vi "Test_DIGIT_5122_Standalone.vi"(8 "error in (no error)":errorcluster, 11 "Use Software Trigger":bool=TRUE) -> (0 "error out":errorcluster)   [LabVIEW 2015]
doc: "This VI inits a waveform generation session for AWG-5421. This is a basic example that shows how to setup the board in order to generate waveforms according to a script. \nBy default this configuration uses one channel CH0, and one script trigger ScriptTrigger0. The ScriptTrigger0 is waiting for an external trigger : i.e. a digital Edge on pin PFI 0 by default.\n\nThere are various options for the script to be used. Consult the Script control help for more information on configuring the example for specific scripts."
uses:
  controls/DIGIT_5122_Inputs.ctl
  <instrlib>/niScope/Controls/niScope trigger source.ctl
  controls/DATA_Inputs.ctl
  controls/SOFTWARE_Inputs.ctl
  <instrlib>/niScope/Configure/Trigger/niScope Configure Trigger Edge.vi
  <instrlib>/niScope/Configure/Trigger/niScope Configure Trigger Immediate.vi
  <instrlib>/niScope/Acquire/Fetch/niScope Multi Fetch Binary 16.vi
panel:
  out "wfm info":T1(array[cluster])
  in  "Number of Acquisitions":i32=2
  in  "Accum Number":i16
  out "ASCII Character":string="T"
  in  "SOFTWARE Inputs":T2={"Application Directory"=path "D:/S.O.F.T.S/LABVIEW/PIL", "Data Path"=path "D:/PIRENEA/DATA", "XML Path"=path "D:/PIRENEA/DATA", "XML File Filter"="*.xml", "XML Saved Path"=path "D:/S.O.F.T.S/LABVIEW/PIL/resources", "Excit Scripts Path"=path "D:/PIRENEA/EXCIT_SCRIPTS", "Excit Scripts File Filter"="*.txt", "Excit Waveforms Path"=path "D:/PIRENEA/EXCIT_WFMS", "Excit Waveforms File Filter"="*.bin", "Timing Scripts Path"=path "D:/PIRENEA/TIMING_SCRIPTS", "Timing Scripts File Filter"="*.txt", "Timing Waveforms Path"=path "D:/PIRENEA/TIMING_WFMS", "Timing Waveforms File Filter"="*.bin", "Trapping Waveforms Path"=path "D:/PIRENEA/TRAPPING_WFMS", "Trapping Waveforms File Filter"="*.bin"} caption="EXCIT Paths"
  out "Graphe":ext[][](graph)
  out "acquisition status":i32
  in  "DATA Inputs":T3={"Record Length"=100000, "Sample Rate"=10000000.0, "Data Type"=0, "Vertical Range"=10.0, "Acquisition Duration"=10.0} {"Vertical Range" items=["0.2"=0.2, "0.4"=0.4, "1"=1.0, "2"=2.0, "4"=4.0, "10"=10.0]; "Data Type" items=["I16", "DBL"]; "Sample Rate" items=["1 MHz"=1000000.0, "2 MHz"=2000000.0, "5 MHz"=5000000.0, "10 MHz"=10000000.0, "20 MHz"=20000000.0, "25 MHz"=25000000.0, "50 MHz"=50000000.0, "100 MHz"=100000000.0]}
  in  "DIGIT 5122 Inputs":T4={"Sample Rate"=10000.0, "Resource Name"="DIGIT_5122", "Channel Name"="0", "Trigger Source"="VAL_EXTERNAL", "Vertical Range"=10.0, "Trigger Level"=3.0} {"Trigger Level" format="%.2f"; "Vertical Range" format="%.2f"; "Sample Rate" step=65535.0 format="%#_3p"}
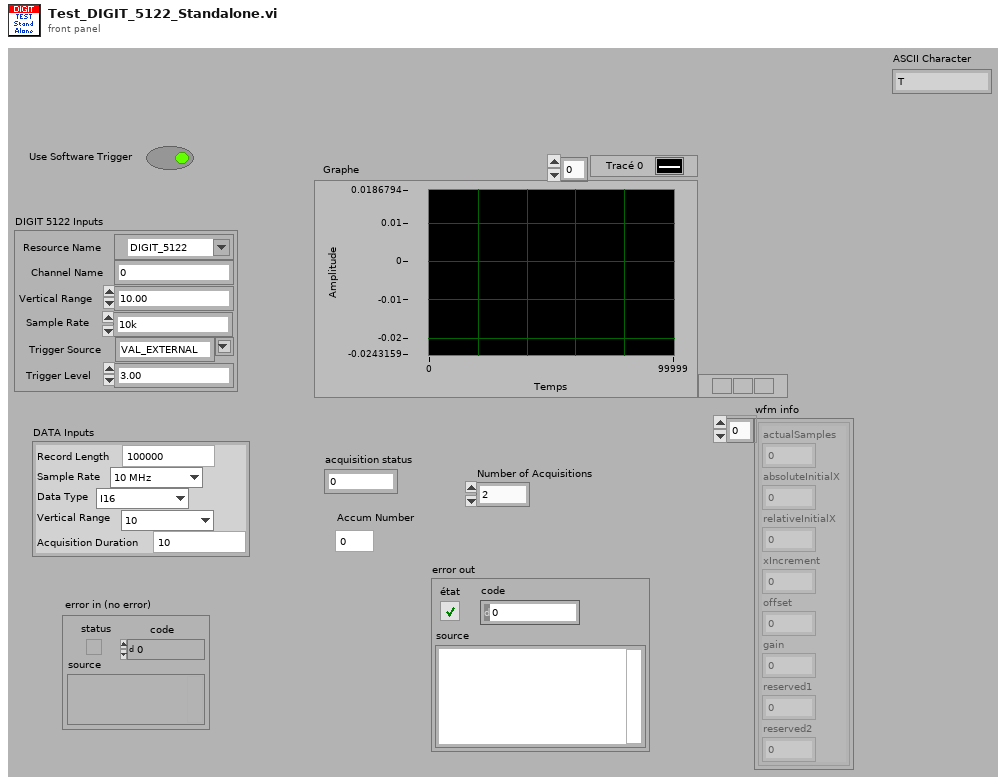
[diagram p1: front panel]
types:
  T1 = cluster{"actualSamples":i32, "absoluteInitialX":dbl, "relativeInitialX":dbl, "xIncrement":dbl, "offset":dbl, "gain":dbl, "reserved1":dbl, "reserved2":dbl}[]
  T2 = typedef "SOFTWARE_Inputs.ctl" = cluster{"Application Directory":path, "Data Path":path, "XML Path":path, "XML File Filter":string, "XML Saved Path":path, "Excit Scripts Path":path, "Excit Scripts File Filter":string, "Excit Waveforms Path":path, "Excit Waveforms File Filter":string, "Timing Scripts Path":path, "Timing Scripts File Filter":string, "Timing Waveforms Path":path, "Timing Waveforms File Filter":string, "Trapping Waveforms Path":path, "Trapping Waveforms File Filter":string}
  T3 = typedef "DATA_Inputs.ctl" = cluster{"Record Length":i32, "Sample Rate":dbl, "Data Type":u8, "Vertical Range":dbl, "Acquisition Duration":dbl}
  T4 = typedef "DIGIT_5122_Inputs.ctl" = cluster{"Sample Rate":dbl, "Resource Name":refnum<k15>, "Channel Name":string, "Trigger Source":T5, "Vertical Range":dbl, "Trigger Level":dbl}
  T5 = typedef "niScope trigger source.ctl" = string
  T6 = enum16{"open", "replace", "create", "open or create", "replace or create", "replace or create with confirmation"}
  T7 = cluster{"actualSamples":i32, "absoluteInitialX":dbl, "relativeInitialX":dbl, "xIncrement":dbl, "offset":dbl, "gain":dbl, "reserved1":dbl, "reserved2":dbl}
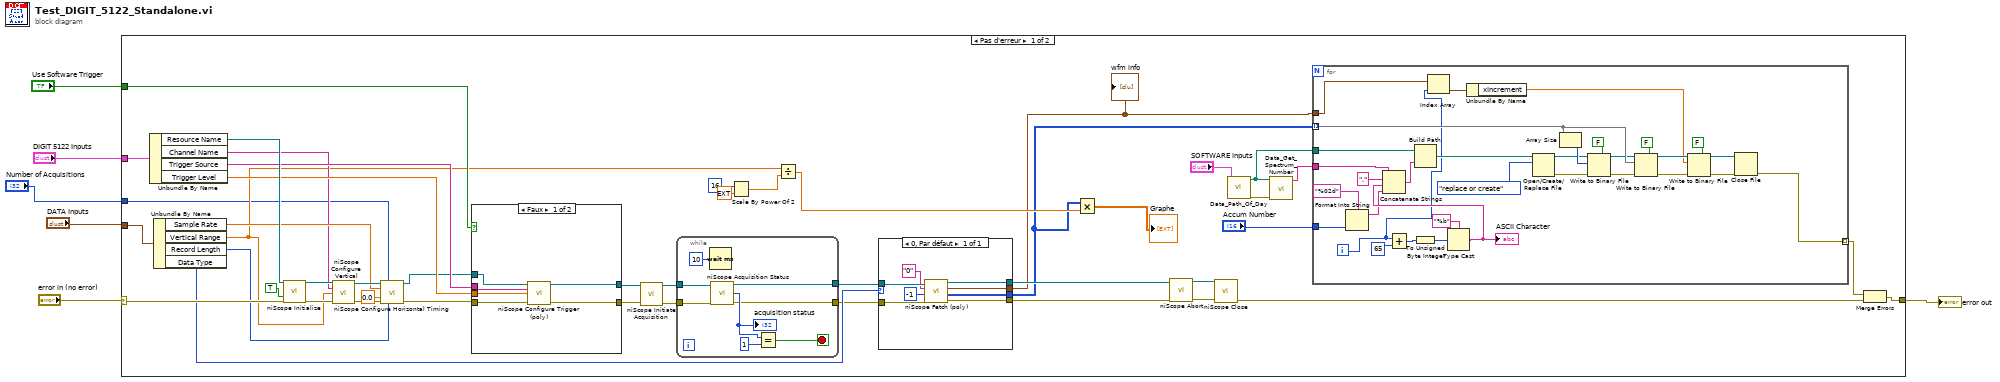
[diagram p0: block diagram]
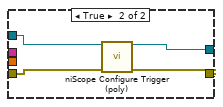
[diagram p2: hidden frame]
diagram:
  n1 = case shown="Pas d'erreur" "error in (no error)" {
    selector: "error in (no error)" -> [w47 w111]
    tunnel: [w26 w111] -> w3
    tunnel: "Use Software Trigger" -> [w52 _]
    tunnel: "DIGIT 5122 Inputs" -> [w51 _]
    tunnel: "DATA Inputs" -> [w50 _]
    tunnel: "Number of Acquisitions" -> [w9 _]
    frame No Error {
      n2 = Unbundle By Name(w51) -> ("Resource Name"=w49:refnum<k15>, "Channel Name"=w33:string, "Trigger Source"=w40:T5, "Trigger Level"=w41:dbl)
      n3 = Unbundle By Name(w50) -> ("Sample Rate"=w37:dbl, "Vertical Range"=w15:dbl, "Record Length"=w42:i32, "Data Type"=w22:u8)
      n4 = call <instrlib>:"niScope Initialize.vi"("resource name"=w49, "reset device"=TRUE, "error in"=w47) -> ("instrument handle"=w46:refnum<k15>, "error out"=w45:errorcluster)  [unwired: 11 in]
      n5 = call <instrlib>:"niScope Configure Vertical.vi"("instrument handle"=w46, "channels"=w33, "vertical range"=w15, "error in"=w45) -> ("instrument handle out"=w44:refnum<k15>, "error out"=w43:errorcluster)  [unwired: 10 in]
      n6 = call <instrlib>:"niScope Configure Horizontal Timing.vi"("instrument handle"=w44, "number of records"=w9, "min sample rate"=w37, "reference position"=0.0, "error in"=w43, "min record length"=w42) -> ("instrument handle out"=w24:refnum<k15>, "error out"=w23:errorcluster)  [unwired: 8 in]
      n7 = case shown="Faux" w52 {
        tunnel: [w94 w100] -> w39
        tunnel: [w93 w99] -> w38
        tunnel: w41 -> [w98 _]
        tunnel: w40 -> [w97 _]
        tunnel: w24 -> [w96 w102]
        tunnel: w23 -> [w95 w101]
        frame False {
          n8 = call-poly <instrlib>:"niScope Configure Trigger (poly).vi"("instrument handle"=w96, "trigger source"=w97, "trigger level"=w98, "error in"=w95) -> ("instrument handle out"=w94:refnum<k15>, "error out"=w93:errorcluster)  [unwired: 10 in]
        }
        frame True {
          n9 = call-poly <instrlib>:"niScope Configure Trigger (poly).vi"("instrument handle"=w102, "error in"=w101) -> ("instrument handle out"=w100:refnum<k15>, "error out"=w99:errorcluster)  [unwired: 12 in]
        }
      }
      n10 = call <instrlib>:"niScope Initiate Acquisition.vi"("instrument handle"=w39, "error in"=w38) -> ("instrument handle out"=w36:refnum<k15>, "error out"=w35:errorcluster)  [unwired: 12 in]
      n11 = while {
        tunnel: w36 -> [w107]
        tunnel: w35 -> [w106]
        tunnel: [w105] -> w34
        tunnel: [w104] -> w10
        stop <- w108 stop-if-true
        n12 = Wait (ms)(milliseconds to wait=u32 10 ("attente (ms)")) -> ()  [unwired: 1 out]
        n13 = call <instrlib>:"niScope Acquisition Status.vi"("instrument handle"=w107, "error in"=w106) -> ("instrument handle out"=w105:refnum<k15>, "acquisition status"=w110:i32, "error out"=w104:errorcluster)  [unwired: 11 in]
        "acquisition status" <- w110
        n14 = Equal?(x=w110, y=1) -> (x = y?=w108:bool)
      }
      n15 = Scale By Power Of 2(n=i16 16, x=ext 1.0) -> (x*2^n=w12:ext)
      n16 = Divide(x=w15, y=w12) -> (x/y=w17:ext)
      n17 = case shown="0, Par défaut" w22 {
        tunnel: w34 -> [w60]
        tunnel: w10 -> [w59]
        tunnel: [w57] -> w21
        tunnel: [w56] -> w20
        tunnel: [w55] -> w16
        tunnel: [w54] -> w8
        frame 0, Default {
          n18 = call-poly <instrlib>:"niScope Fetch (poly).vi"("error in"=w59, "numSamples"=-1, "channels"="0", "instrument handle"=w60) -> ("error out"=w56:errorcluster, "wfm"=w55:i16[][], "wfm info"=w54:T1, "instrument handle out"=w57:refnum<k15>)  [unwired: 4 in]
        }
      }
      "wfm info" <- w8
      n19 = Multiply(x=w16, y=w17) -> (x*y=→"Graphe":ext[][])
      n20 = call <instrlib>:"niScope Abort.vi"("instrument handle"=w21, "error in"=w20) -> ("instrument handle out"=w18:refnum<k15>, "error out"=w19:errorcluster)  [unwired: 12 in]
      n21 = call <instrlib>:"niScope Close.vi"("instrument handle"=w18, "error in"=w19) -> ("error out"=w28:errorcluster)  [unwired: 13 in]
      n22 = call "Data_Path_Of_Day.vi"("SOFTWARE Inputs"="SOFTWARE Inputs") -> ("error out"=w32:errorcluster, "Path of the Day"=w29:path)  [unwired: 9 in]
      n23 = call "Data_Get_Spectrum_Number.vi"("error in (no error)"=w32, "Path of the Day"=w29) -> ("Next Spectrum Number"=w30:string)  [unwired: 7 in, 2 out]
      n24 = for {
        tunnel: w16 -> [w76] mode=indexing
        tunnel: w30 -> [w88]
        tunnel: w29 -> [w83]
        tunnel: [w80] -> w27 mode=indexing
        tunnel: "Accum Number" -> [w79]
        tunnel: w8 -> [w63]
        i -> [w62]
        n25 = Format Into String(format string="%02d" ("chaîne de format"), w79) -> (resulting string=w77:string)  [unwired: 2 in, 1 out]
        n26 = Add(x=w62, y=i16 65) -> (x+y=w89:i32)
        n27 = To Unsigned Byte Integer(number=w89) -> (unsigned 8bit integer=w90:u8)
        n28 = Index Array(array=w63, index=w62) -> (element=w61:T7)
        n29 = Type Cast(type="%b", x=w90) -> (*(type *) &x=w86:string)
        "ASCII Character" <- w86
        n30 = Concatenate Strings(w88, "." ("chaîne"), w86, w77) -> (w82:string)
        n31 = Build Path(base path=w83, name or relative path=w82) -> (appended path=w81:path)
        n32 = Unbundle By Name(w61) -> ("xIncrement"=w64:dbl)
        n33 = Open/Create/Replace File(file path (use dialog)=w81, operation (0:open)=T6."replace or create" ("opération (0 : open)")) -> (refnum out=w74:refnum<file>, error out=w73:errorcluster)  [unwired: 4 in, 1 out]
        n34 = Array Size(array=w76) -> (size(s)=w75:i32)
        n35 = Write to Binary File(file (use dialog)=w74, data=w75, error in=w73, 5:FALSE ("ajouter une taille de tableau ou de chaîne ? (V)")) -> (refnum out=w70:refnum<file>, error out=w71:errorcluster)  [unwired: 2 in, 1 out]
        n36 = Write to Binary File(file (use dialog)=w70, data=w76, error in=w71, 5:FALSE ("ajouter une taille de tableau ou de chaîne ? (V)")) -> (refnum out=w68:refnum<file>, error out=w69:errorcluster)  [unwired: 2 in, 1 out]
        n37 = Write to Binary File(file (use dialog)=w68, data=w64, error in=w69, 5:FALSE ("ajouter une taille de tableau ou de chaîne ? (V)")) -> (refnum out=w66:refnum<file>, error out=w65:errorcluster)  [unwired: 2 in, 1 out]
        n38 = Close File(refnum=w66, error in=w65) -> (error out=w80:errorcluster)  [unwired: 1 out]
      }
      n39 = Merge Errors(w27, w28) -> (w26:errorcluster)
    }
    frame Error {
    }
  }
  "error out" <- w3
